vi "Match Multiple Pattern_csm.vi"(7 "delimiter (|)":string="|", 8 "offset (0)":i32, 10 "regular expression":string, 11 "string":string) -> (0 "Found?":bool, 1 "after substring":string, 2 "match substring":string, 3 "before substring":string, 4 "pattern matched":string)   [LabVIEW 2017, in "API String Arguments Support.lvlib"]
doc: "Searches for <b>regular expression</b> sequentially in <b>string</b> beginning at <b>offset</b>. If the function finds the first match, it splits <b>string</b> into three substrings.\n\nAs a supplement to <b>Match Pattern Function</b>, <b>regular expression</b> can include mutiple regular expression, and they are separated by <b>delimiter</b>."
uses:
  API String Arguments Support.lvlib
  <userlib>/_NEVSTOP/Communicable State Machine(CSM)/Communicable State Machine.lvlib
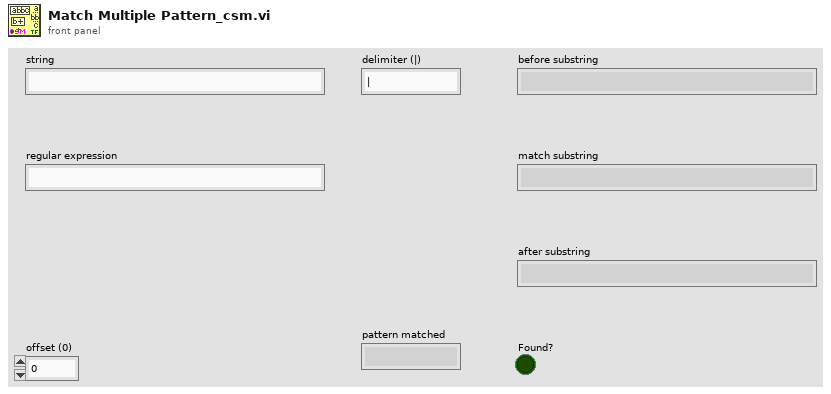
[diagram p1: front panel]
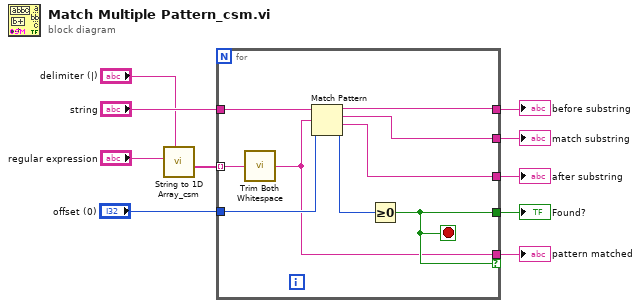
[diagram p0: block diagram]
diagram:
  n1 = call <userlib>:"String to 1D Array_csm.vi"("delimiter (Tab)"="delimiter (|)", "string"="regular expression") -> ("Array of Strings"=w1:string[])  [unwired: 9 in]
  n2 = for {
    tunnel: "offset (0)" -> [w18]
    tunnel: [w15] -> w6
    tunnel: [w12] -> w5
    tunnel: "string" -> [w19]
    tunnel: [w17] -> w8
    tunnel: w1 -> [w13] mode=indexing
    tunnel: [w16] -> w7
    tunnel: [w11] -> w2 if=w12
    stop <- w12 stop-if-true
    n3 = call <userlib>:"Trim Both Whitespace.vi"("string"=w13) -> ("trimmed string"=w11:string)  [unwired: 1 in]
    n4 = Match Pattern(string=w19, regular expression=w11, offset (0)=w18) -> (before substring=w17:string, match substring=w16:string, after substring=w15:string, offset past match=w14:i32)
    n5 = Greater Or Equal To 0?(x=w14) -> (x >= 0?=w12:bool)
  }
  "before substring" <- w8
  "match substring" <- w7
  "after substring" <- w6
  "Found?" <- w5
  "pattern matched" <- w2
